vi "Prepare SUBACK Response.vi"(8 "error in (no error)":errorcluster, 10 "Return Codes":T1[](array[typedef]), 11 "SUBSCRIBE in":refnum<class "SUBSCRIBE.lvclass">) -> (0 "error out":errorcluster, 1 "response prepared?":bool, 2 "SUBACK response":refnum<class "SUBACK.lvclass">, 3 "SUBSCRIBE out":refnum<class "SUBSCRIBE.lvclass">)   [LabVIEW 2013, in "MQTT_Control_Packets.lvlib" / "SUBSCRIBE.lvclass"]
uses:
  SUBSCRIBE.lvclass
  SUBACK/SUBACK.lvclass
  SUBACK/Subscription Success Code.ctl
  ControlPacket/QualityOfService -- enum.ctl
  ControlPacket/ControlPacket.lvclass/ControlPacket.ctl
  ControlPacket/ControlPacket.lvclass
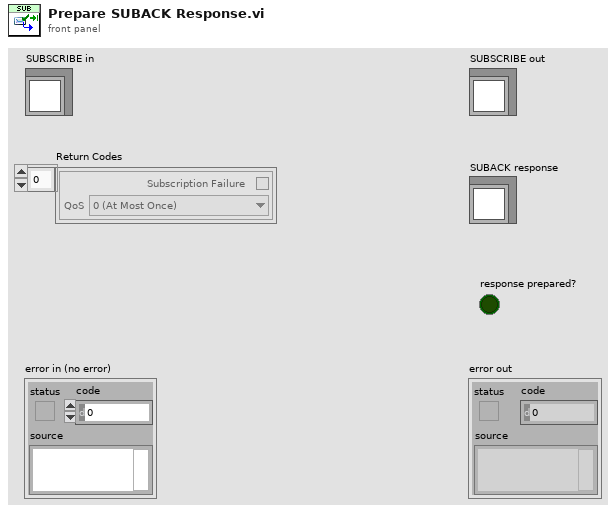
[diagram p1: front panel]
types:
  T1 = typedef "MQTT_Control_Packets.lvlib/SUBACK.lvclass/Subscription Success Code.ctl" = cluster{"Subscription Failure":bool, "QoS":T2}
  T2 = typedef "MQTT_Control_Packets.lvlib/ControlPacket.lvclass/QualityOfService -- enum.ctl" = enum16{"0 (At Most Once)", "1 (At Least Once)", "2 (Exactly Once)"}
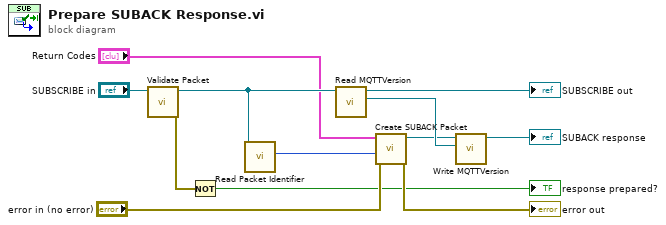
[diagram p0: block diagram]
diagram:
  n1 = call "Validate Packet.vi"("ControlPacket in"="SUBSCRIBE in") -> ("error out"=w6:errorcluster, "ControlPacket out"=w3:refnum<class "SUBSCRIBE.lvclass">)  [unwired: 9 in]
  n2 = Not(x=w6) -> (.not. x?=→"response prepared?":bool)
  n3 = call "Read Packet Identifier.vi"("ControlPacket in"=w3) -> ("Packet Identifier"=w2:u16)  [unwired: 9 in, 1 out]
  n4 = call "Read MQTTVersion.vi"("ControlPacket in"=w3) -> ("MQTTVersion"=w12:refnum<class "MQTTVersion.lvclass">, "ControlPacket out"=→"SUBSCRIBE out":refnum<class "SUBSCRIBE.lvclass">)  [unwired: 9 in]
  n5 = call "Create SUBACK Packet.vi"("error in (no error)"="error in (no error)", "Packet ID"=w2, "Return Codes"="Return Codes") -> ("error out"=→"error out":errorcluster, "SUBACK"=w10:refnum<class "SUBACK.lvclass">)  [unwired: 6 in, 1 out]
  n6 = call "Write MQTTVersion.vi"("MQTTVersion"=w12, "ControlPacket in"=w10) -> ("ControlPacket out"=→"SUBACK response":refnum<class "SUBACK.lvclass">)  [unwired: 9 in]
